vi "Decimation Channel.vi"(6 "Embedded Data Logger Channel Group Name":string, 7 "Embedded Data Logger File Name":string, 8 "error in":errorcluster, 10 "Decimation":dbl, 11 "Embedded Data Logger System Tests in":refnum<class "Embedded Data Logger Windows System Tests.lvclass">) -> (0 "error out":errorcluster, 3 "Embedded Data Logger System Tests out":refnum<class "Embedded Data Logger Windows System Tests.lvclass">)   [LabVIEW 2027, in "Embedded Data Logger Windows System Tests.lvclass"]
uses:
  Embedded Data Logger Windows System Tests.lvclass
  C:/Program Files/National Instruments/LabVIEW 2027/vi.lib/NI/VeriStand Custom Device Testing Tools/VeriStandTestCase/VeriStandTestCase.lvclass
  <vilib>/NI VeriStand/Execution/Workspace/NI VeriStand - Set Single Channel Value.vi
  <vilib>/NI VeriStand/Execution/Workspace/NI_VS Workspace ExecutionAPI.lvlib
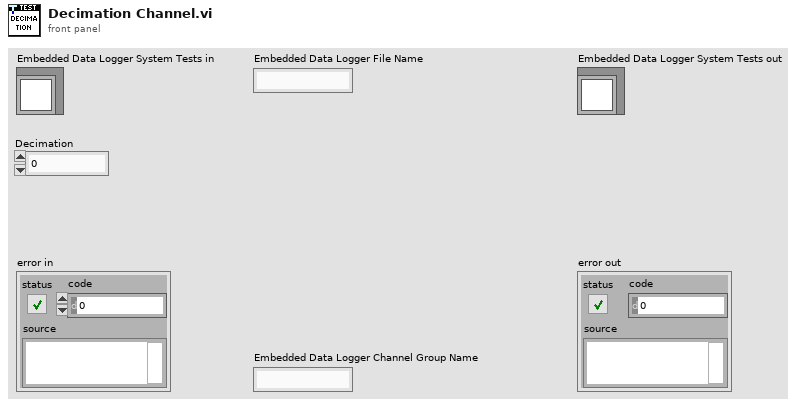
[diagram p1: front panel]
types:
  T1 = typedef "NI_VS Workspace ExecutionAPI.lvlib/WorkspaceAPI.ctl" = refnum<k39>
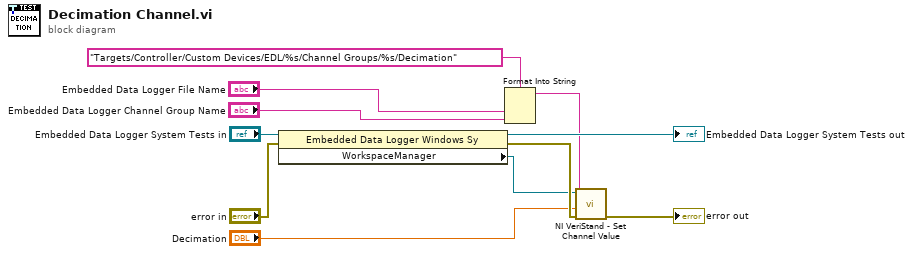
[diagram p0: block diagram]
diagram:
  n1 = property class="Embedded Data Logger Windows Sy"(reference="Embedded Data Logger System Tests in", error in="error in") -> (reference out=→"Embedded Data Logger System Tests out":refnum<class "Embedded Data Logger Windows System Tests.lvclass">, error out=w9:errorcluster, "WorkspaceManager"=w8:T1)
  n2 = Format Into String(format string="Targets/Controller/Custom Devices/EDL/%s/Channel Groups/%s/Decimation" ("Channel"), "Embedded Data Logger File Name", "Embedded Data Logger Channel Group Name") -> (resulting string=w5:string)  [unwired: 2 in, 1 out]
  n3 = call-poly <vilib>:"NI VeriStand - Set Channel Value.vi"("error in (no error)"=w9, "Value"="Decimation", "Channel"=w5, "WorkspaceManager in"=w8) -> ("error out"=→"error out":errorcluster)  [unwired: 6 in, 1 out]
